vi "Configure Modulation Format Test Pattern.vi"(8 "error in (no error)":errorcluster {"code" format="%.0x"}, 9 "TestPattern (Standard1011)":i32(ring) items=["Standard1011", "Standard511", "Standard Calibration", "Standard Inbound1011", "Standard Inbound511", "Standard Inbound Calibration", "None"], 10 "ModulationType (apco2 5c 4fm)":i32(ring) items=["apco2 5c 4fm", "dmr", "None"], 11 "instrument handle":refnum<k15>) -> (0 "error out":errorcluster {"code" format="%.0x"}, 3 "instrument handle out":refnum<k15>)   [LabVIEW 2009, in "Keysight XSAn.lvlib"]
doc: "Configure modulation format test pattern."
uses:
  <instrlib>/Keysight XSAn/Keysight XSAn.lvlib
  AgXSAn.dll
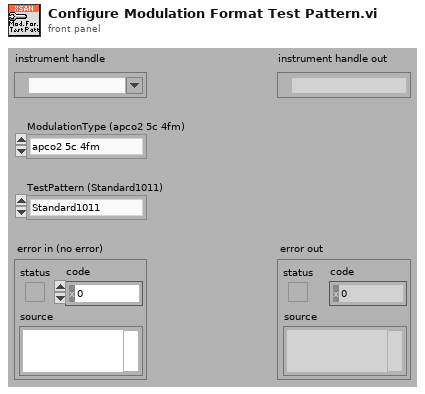
[diagram p1: front panel]
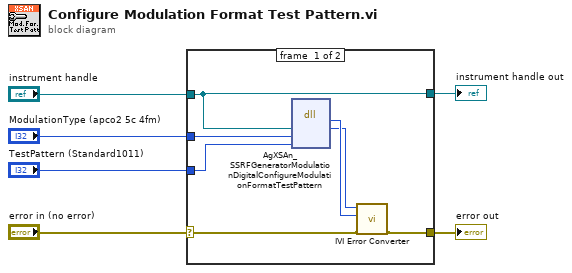
[diagram p0: block diagram]
diagram:
  n1 = case shown="No Error" "error in (no error)" {
    selector: "error in (no error)" -> [w8 w15]
    tunnel: [w9 w15] -> w6
    tunnel: "instrument handle" -> [w7 w14]
    tunnel: "ModulationType (apco2 5c 4fm)" -> [w13 _]
    tunnel: "TestPattern (Standard1011)" -> [w12 _]
    tunnel: [w7 w14] -> w1
    frame #0 {
      n2 = dll-call lib="AgXSAn**.dll" fn="AgXSAn_SSRFGeneratorModulationDigitalConfigureModulationFormatTestPattern"("Vi"=w7, "ModulationType"=w13, "TestPattern"=w12) -> (w11:i32, "Vi"=w10:u32)  [unwired: 5 in, 2 out]
      n3 = call <instrlib>:"IVI Error Converter.vi"("error in (no error)"=w8, "IVI error code (0)"=w11, "instrument handle"=w10) -> ("error out"=w9:errorcluster)  [unwired: 7 in, 1 out]
    }
    frame #1 {
    }
  }
  "error out" <- w6
  "instrument handle out" <- w1
